vi "Scale.vi"(10 "Sensativity":dbl, 11 "Band Power (dB SPL)":dbl[](array[numeric])) -> (3 "SPL Scaled":dbl[](array[numeric]))   [LabVIEW 2024]
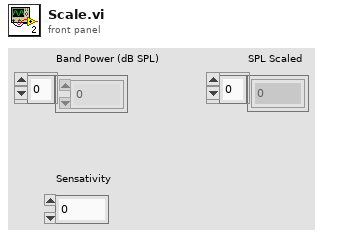
[diagram p1: front panel]
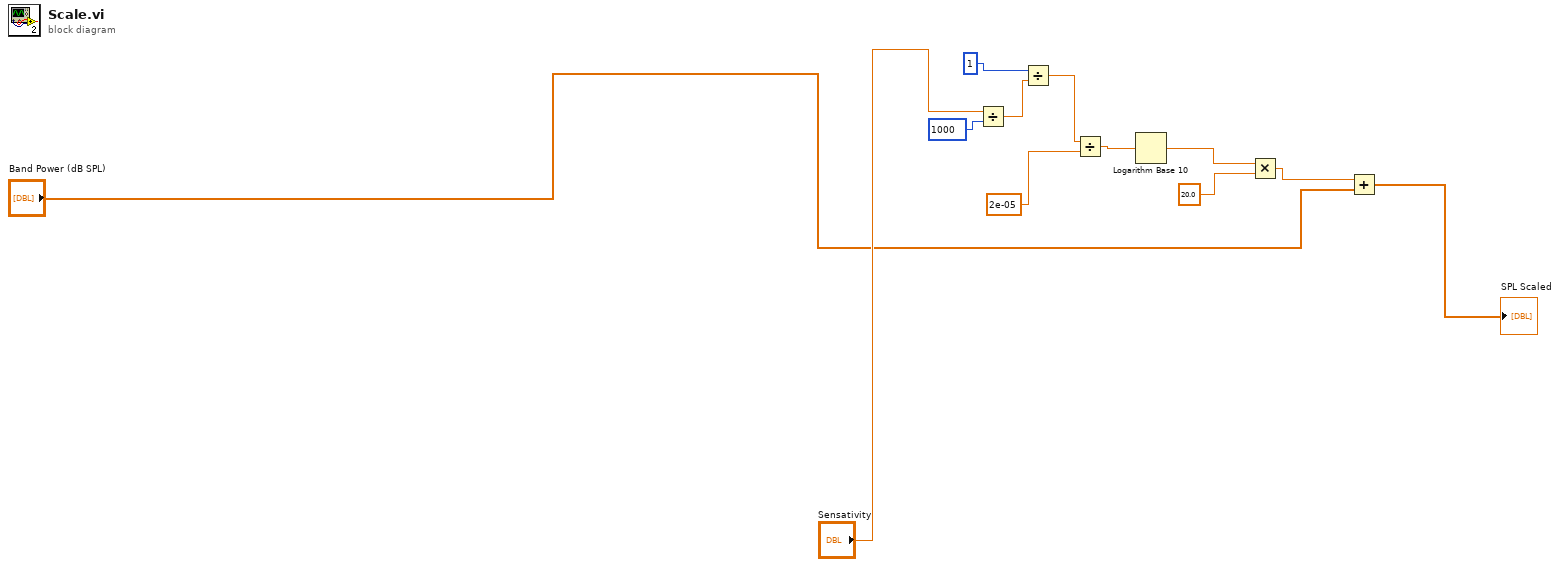
[diagram p0: block diagram]
diagram:
  n1 = Divide(x="Sensativity", y=1000) -> (x/y=w6:dbl)
  n2 = Divide(x=1, y=w6) -> (x/y=w5:dbl)
  n3 = Divide(x=w5, y=2e-05) -> (x/y=w4:dbl)
  n4 = Logarithm Base 10(1:w4) -> (0:w2:dbl)
  n5 = Multiply(x=w2, y=20.0) -> (x*y=w1:dbl)
  n6 = Add(x=w1, y="Band Power (dB SPL)") -> (x+y=→"SPL Scaled":dbl[])
